vi "setup led serial.vi"(8 "error in (no error)":errorcluster, 11 "Teensy Serial Port":refnum<visa-resource-name>) -> (0 "error out":errorcluster, 2 "OK":bool, 3 "Teensy Serial Port":refnum<visa-resource-name>)   [LabVIEW 2013]
uses:
  <vilib>/Instr/_visa.llb/VISA Flush IO Buffer Mask.ctl
  <vilib>/Instr/_visa.llb/VISA Set IO Buffer Mask.ctl
  <vilib>/Instr/_visa.llb/VISA Configure Serial Port (Instr).vi
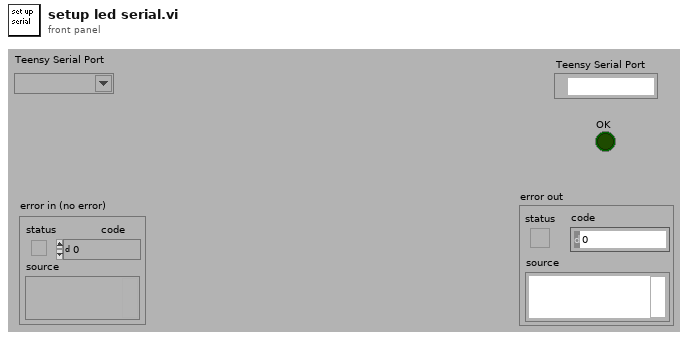
[diagram p1: front panel]
types:
  T1 = typedef "VISA Set IO Buffer Mask.ctl" = u16
  T2 = enum16{"R - open file for Reading", "W - open file for Writing", "S - send bytes", "F - fetch bytes", "B - begin experiment", "E - end experiment", "N - set number of bits per frame", "I - get info", "Q - Quiet (only error msgs)", "L - Loud (acknowledge all)", "T - set stimulus state", "Y - ready to start experiment", "H - useless Help message"}
  T3 = typedef "VISA Flush IO Buffer Mask.ctl" = u16
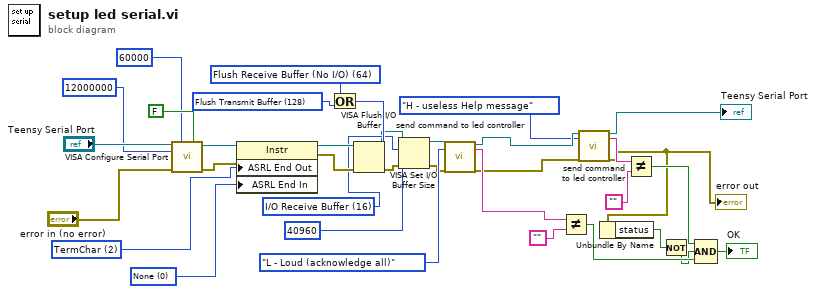
[diagram p0: block diagram]
diagram:
  w2 = u16 0 items=["None", "Last Bit", "TermChar"] ("Serial Settings:End Mode for Reads")
  w6 = T1 16 items=["I/O Receive Buffer"=16, "I/O Transmit Buffer"=32, "I/O Receive and Transmit Buffer"=48] ("Mask")
  w24 = T3 128 items=["Flush Receive Buffer"=16, "Write Transmit Buffer to Device"=32, "Flush Receive Buffer (No I/O)"=64, "Flush Transmit Buffer"=128] ("x .or. y?")
  w26 = T3 64 items=["Flush Receive Buffer"=16, "Write Transmit Buffer to Device"=32, "Flush Receive Buffer (No I/O)"=64, "Flush Transmit Buffer"=128] ("Mask")
  w29 = u16 2 items=["None", "Last Bit", "TermChar", "Break"] ("Serial Settings:End Mode for Writes")
  n1 = call-poly "VISA Configure Serial Port"("VISA resource name"="Teensy Serial Port", "timeout (10sec)"=u32 60000, "Enable Termination\nChar (T)"=FALSE ("Enable Termination\nChar (T)"), "baud rate (9600)"=u32 12000000, "error in (no error)"="error in (no error)") -> ("VISA resource name out"=w31:refnum<visa-resource-name>, "error out"=w30:errorcluster)  [unwired: 9 in]
  n2 = property class="Instr"(reference=w31, error in=w30, "ASRL End Out"=w29, "ASRL End In"=w2) -> (reference out=w27:refnum<visa-resource-name>, error out=w28:errorcluster)
  n3 = Or(x=w26, y=w24) -> (x .or. y?=w25:T3)
  n4 = VISA Flush I/O Buffer(VISA resource name=w27, mask (16)=w25, error in (no error)=w28) -> (VISA resource name out=w4:refnum<visa-resource-name>, error out=w8:errorcluster)
  n5 = VISA Set I/O Buffer Size(VISA resource name=w4, mask (16)=w6, size (4096)=u32 40960, error in (no error)=w8) -> (VISA resource name out=w3:refnum<visa-resource-name>, error out=w7:errorcluster)
  n6 = call "send command to led controller.vi"("Teensy Serial Port"=w3, "Command"=T2."L - Loud (acknowledge all)", "error in"=w7) -> ("teensy serial port out"=w13:refnum<visa-resource-name>, "response"=w21:string, "error out"=w14:errorcluster)  [unwired: 11 in, 3 out]
  n7 = Not Equal?(x=w21, y="") -> (x != y?=w16:bool)
  n8 = call "send command to led controller.vi"("Teensy Serial Port"=w13, "Command"=T2."H - useless Help message", "error in"=w14) -> ("teensy serial port out"=→"Teensy Serial Port":refnum<visa-resource-name>, "response"=w20:string, "error out"=w9:errorcluster)  [unwired: 11 in, 3 out]
  "error out" <- w9
  n9 = Unbundle By Name(w9) -> ("status"=w11:bool)
  n10 = Not Equal?(x=w20, y="") -> (x != y?=w17:bool)
  n11 = Not(x=w11) -> (.not. x?=w10:bool)
  n12 = Compound Arithmetic op=AND(w17, w10, w16) -> (→"OK":bool)
